vi "Write Current_Share.vi"(8 "error in":errorcluster, 10 "Current_Sharing":bool, 11 "69X_79X in":refnum<class "7976A.lvclass">) -> (0 "error out":errorcluster, 3 "69X_79X out":refnum<class "7976A.lvclass">)   [LabVIEW 2019, in "7976A.lvlib" / "7976A.lvclass"]
uses:
  Library/7976A.lvclass
  builds/Instruments/PowerSupply.lvlibp/Library/PowerSupply.lvclass
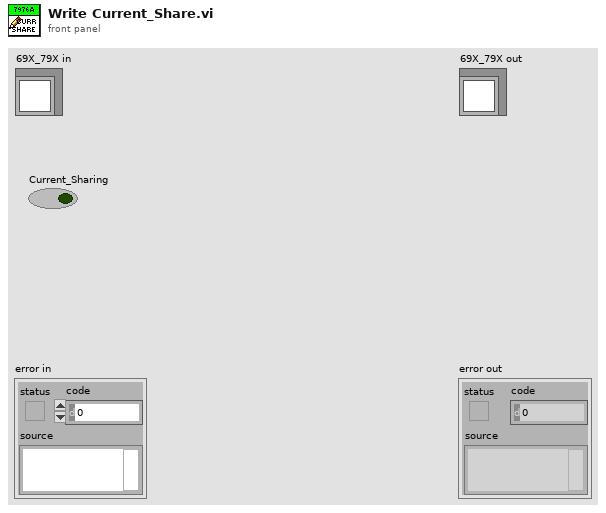
[diagram p1: front panel]
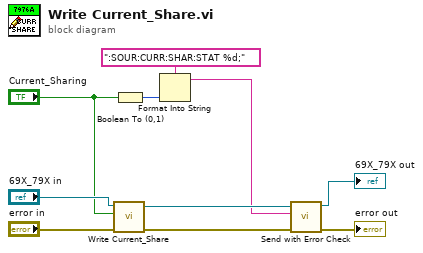
[diagram p0: block diagram]
diagram:
  n1 = call-parent "Write Current_Share.vi"("error in"="error in", "Current_Sharing"="Current_Sharing", "PowerSupply in"="69X_79X in") -> ("error out"=w3:errorcluster, "PowerSupply out"=w5:refnum<class "7976A.lvclass">)  [unwired: 7 in]
  n2 = Boolean To (0,1)(Boolean="Current_Sharing") -> (0, 1=w7:i16)
  n3 = Format Into String(format string=":SOUR:CURR:SHAR:STAT %d;", w7) -> (resulting string=w1:string)  [unwired: 2 in, 1 out]
  n4 = call "Send with Error Check.vi"("error in (no error)"=w3, "Command"=w1, "7976A in"=w5) -> ("error out"=→"error out":errorcluster, "7976A out"=→"69X_79X out":refnum<class "7976A.lvclass">)  [unwired: 7 in]
